vi "UI Stop Operation.vi"(8 "error in (no error)":errorcluster, 10 "UI Console MSG In":refnum<class "UI Console MSG.lvclass">, 11 "UI Console in":refnum<class "UI Console.lvclass">) -> (0 "error out":errorcluster, 2 "Stop":bool=TRUE, 3 "UI Console out":refnum<class "UI Console.lvclass">)   [LabVIEW 2024, in "UI Console.lvclass"]
uses:
  UI Console.lvclass
  UI Console MSG/UI Console MSG.lvclass
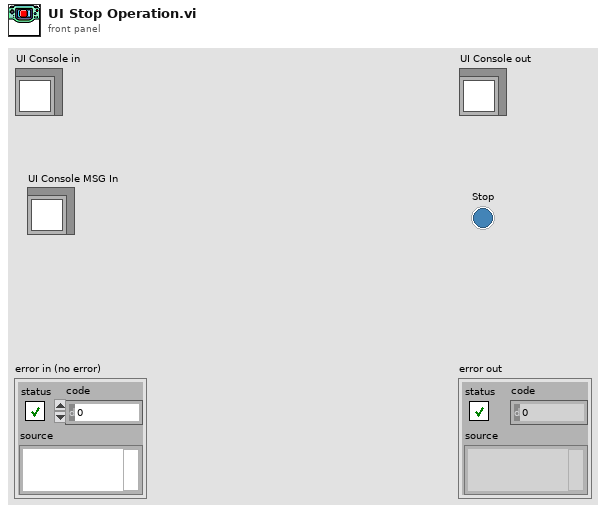
[diagram p1: front panel]
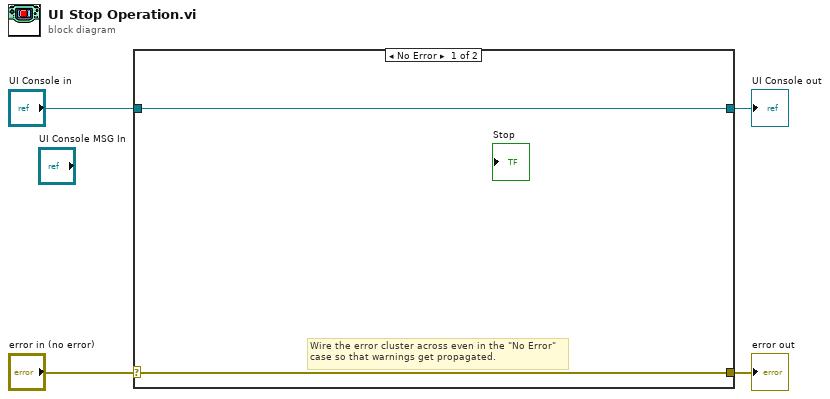
[diagram p0: block diagram]
diagram:
  n1 = case shown="No Error" "error in (no error)" {
    selector: "error in (no error)" -> [w5 w8]
    tunnel: [w5 w8] -> w3
    tunnel: [w6 w7] -> w1
    tunnel: "UI Console in" -> [w6 w7]
    frame No Error {
      # "Wire the error cluster across even in the \"No Error\"\ncase so that warnings get propagated."
    }
    frame Error {
    }
  }
  "error out" <- w3
  "UI Console out" <- w1
